vi "AlliGator Clip Decay for Fit.vi"(8 "Error In":errorcluster, 9 "Min Decay Percentile (0)":dbl, 10 "Max Decay Percentile (1)":dbl=1.0, 11 "Decay in":cluster{"t Array":dbl[], "Value Array":dbl[]}) -> (0 "Error Out":errorcluster, 1 "Index Min":i32, 2 "Index Max":i32, 3 "Clipped Decay out":cluster{"t Array":dbl[], "Value Array":dbl[]}, 4 "# Points":i32)   [LabVIEW 2021, in "AlliGator Decay Analysis.lvlib" / "AlliGator Decay Fit.lvlib"]
doc: "Clips the decay according to the <B>Min</B> and <B>Max Decay Percentile</B> parameters provided.\n\nIf the decay range is [I_min, I_max] and the decay percentiles are (f_min, f_max) in [0, 1], we look for:\n\n- starting from the location of the maximum (presumably the peak location) and moving forward, the point at which:\n\nI_i < I_min + f_max*(I_max - I_min) = F_max\n\n- starting from the last point and moving baclwards, the point at which:\n\nI_i > I_min + f_min*(I_max - I_min) = F_min"
uses:
  AlliGator Decay Fit.lvlib
panel:
  out "XY Graph":cluster{"t Array":dbl[], "Value Array":dbl[]}[](graph)
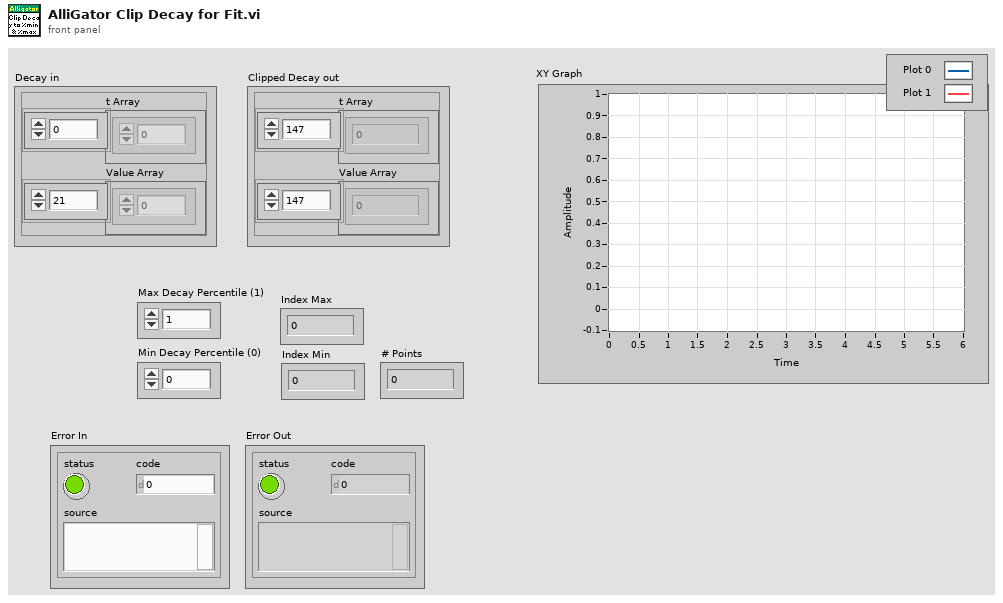
[diagram p1: front panel]
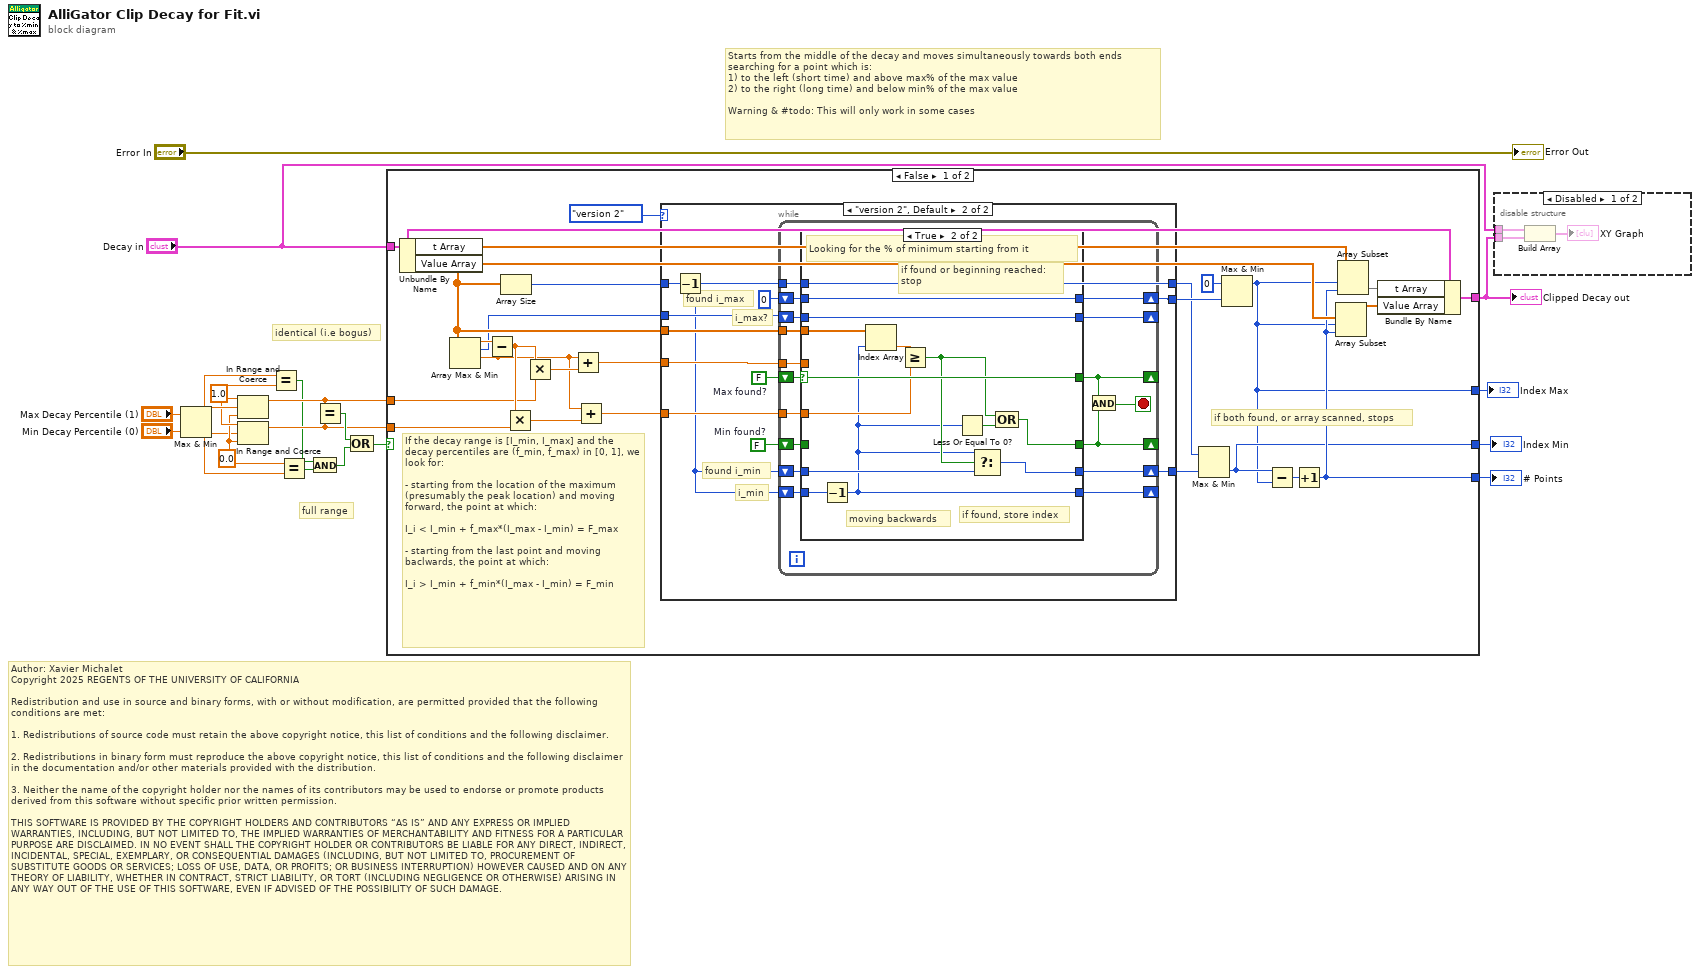
[diagram p0: block diagram]
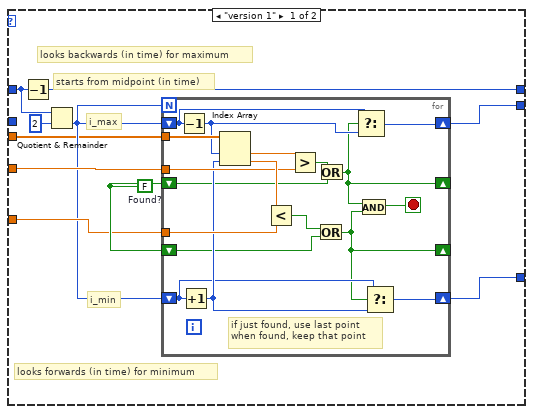
[diagram p2: hidden frame]
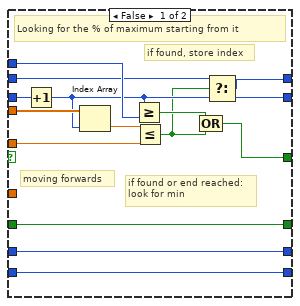
[diagram p3: hidden frame]
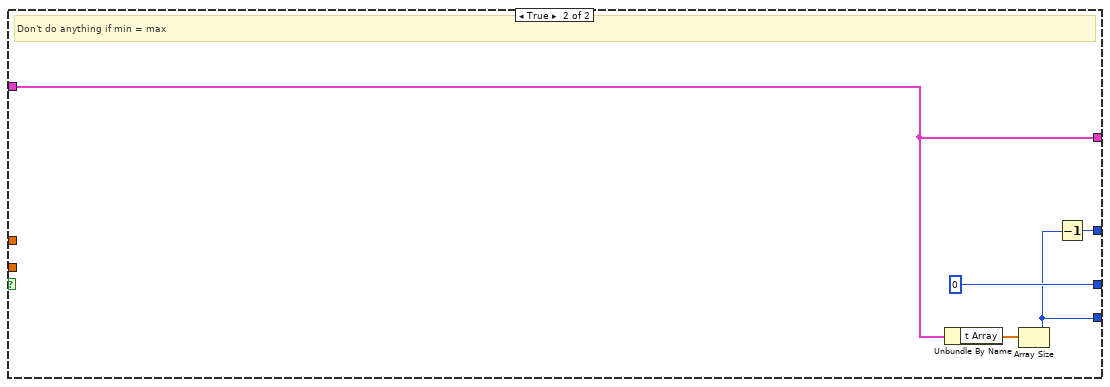
[diagram p4: hidden frame]
diagram:
  w7 = 1.0 ("upper limit")
  w6 = 0.0 ("lower limit")
  # "Author: Xavier Michalet\nCopyright 2025 REGENTS OF THE UNIVERSITY OF CALIFORNIA\n\nRedistribution and use in source and binary forms, with or without modification, are permitted provided that the following conditions are met:\n\n1. Redistributions of source code must retain the above copyright notice, this list of conditions and the following disclaimer.\n\n2. Redistributions in binary form must reproduce the above copyright notice, this list of conditions and the following disclaimer in the documentation and/or other materials provided with the distribution.\n\n3. Neither the name of the copyright holder nor the names of its contributors may be used to endorse or promote products derived from this software without specific prior written permission.\n\nTHIS SOFTWARE IS PROVIDED BY THE COPYRIGHT HOLDERS AND CONTRIBUTORS “AS IS” AND ANY EXPRESS OR IMPLIED WARRANTIES, INCLUDING, BUT NOT LIMITED TO, THE IMPLIED WARRANTIES OF MERCHANTABILITY AND FITNESS FOR A PARTICULAR PURPOSE ARE DISCLAIMED. IN NO EVENT SHALL THE COPYRIGHT HOLDER OR CONTRIBUTORS BE LIABLE FOR ANY DIRECT, INDIRECT, INCIDENTAL, SPECIAL, EXEMPLARY, OR CONSEQUENTIAL DAMAGES (INCLUDING, BUT NOT LIMITED TO, PROCUREMENT OF SUBSTITUTE GOODS OR SERVICES; LOSS OF USE, DATA, OR PROFITS; OR BUSINESS INTERRUPTION) HOWEVER CAUSED AND ON ANY THEORY OF LIABILITY, WHETHER IN CONTRACT, STRICT LIABILITY, OR TORT (INCLUDING NEGLIGENCE OR OTHERWISE) ARISING IN ANY WAY OUT OF THE USE OF THIS SOFTWARE, EVEN IF ADVISED OF THE POSSIBILITY OF SUCH DAMAGE."
  # "identical (i.e bogus)"
  # "full range"
  # "Starts from the middle of the decay and moves simultaneously towards both ends\nsearching for a point which is:\n1) to the left (short time) and above max% of the max value\n2) to the right (long time) and below min% of the max value\n\nWarning & #todo: This will only work in some cases"
  n1 = Max & Min(x="Max Decay Percentile (1)", y="Min Decay Percentile (0)") -> (max(x,y)=w8:dbl, min(x,y)=w5:dbl)
  n2 = In Range and Coerce(upper limit=w7, x=w8, lower limit=w6) -> (coerced(x)=w9:dbl)  [unwired: 1 out]
  n3 = In Range and Coerce(upper limit=w7, x=w5, lower limit=w6) -> (coerced(x)=w10:dbl)  [unwired: 1 out]
  n4 = Equal?(x=w8, y=w7) -> (x = y?=w2:bool)
  n5 = Equal?(x=w6, y=w5) -> (x = y?=w3:bool)
  n6 = And(x=w2, y=w3) -> (x .and. y?=w1:bool)
  n7 = Equal?(x=w9, y=w10) -> (x = y?=w11:bool)
  n8 = Compound Arithmetic op=OR(w11, w1) -> (w4:bool)
  n9 = case shown="False" w4 {
    tunnel: "Decay in" -> [w32 w133]
    tunnel: [w31 w133] -> w17
    tunnel: w9 -> [w26 _]
    tunnel: w10 -> [w25 _]
    tunnel: [w24 w130] -> w16
    tunnel: [w23 0] -> w15
    tunnel: [w22 w129] -> w14
    frame False {
      # "If the decay range is [I_min, I_max] and the decay percentiles are (f_min, f_max) in [0, 1], we look for:\n\n- starting from the location of the maximum\n(presumably the peak location) and moving \nforward, the point at which:\n\nI_i < I_min + f_max*(I_max - I_min) = F_max\n\n- starting from the last point and moving\nbaclwards, the point at which:\n\nI_i > I_min + f_min*(I_max - I_min) = F_min"
      # "if both found, or array scanned, stops"
      n10 = Unbundle By Name(w32) -> ("t Array"=w38:dbl[], "Value Array"=w35:dbl[])
      n11 = Array Max & Min(array=w35) -> (max value=w45:dbl, max index (indices)=w20:i32, min value=w41:dbl)  [unwired: 1 out]
      n12 = Subtract(x=w45, y=w41) -> (x-y=w44:dbl)
      n13 = Array Size(array=w35) -> (size(s)=w30:i32)
      n14 = Multiply(x=w44, y=w25) -> (x*y=w42:dbl)
      n15 = Multiply(x=w44, y=w26) -> (x*y=w43:dbl)
      n16 = Add(x=w41, y=w43) -> (x+y=w40:dbl)
      n17 = Add(x=w41, y=w42) -> (x+y=w39:dbl)
      n18 = case shown="\"version 2\", Default" enum16{"version 1", "version 2"}."version 2" {
        tunnel: w40 -> [w53 w83]
        tunnel: w39 -> [w52 w82]
        tunnel: w35 -> [w50 w81]
        tunnel: [w49 w76] -> w34
        tunnel: w30 -> [w48 w80]
        tunnel: [w47 w75] -> w29
        tunnel: [w46 w74] -> w28
        tunnel: w20 -> [_ w78]
        frame "version 1" {
          w55 = FALSE  # Found?
          # "looks forwards (in time) for minimum"
          # "looks backwards (in time) for maximum"
          # "starts from midpoint (in time)"
          # "i_min"
          # "i_max"
          n19 = Decrement(x=w48) -> (x-1=w46:i32)
          n20 = Quotient & Remainder(x=w48, y=2) -> (floor(x/y)=w51:i32)  [unwired: 1 out]
          n21 = for {
            N: w51 -> [_]
            shift-right: [w66] -> w49
            shift-left: w51 -> [w67]
            shift-right: [w62] -> w47
            shift-left: w51 -> [w61]
            tunnel: w53 -> [w69]
            tunnel: w52 -> [w71]
            tunnel: w50 -> [w73]
            shift-right: [w57] -> _
            shift-left: w55 -> [w60]
            shift-right: [w56] -> _
            shift-left: w55 -> [w59]
            stop <- w58 stop-if-true
            # "if just found, use last point\nwhen found, keep that point"
            n22 = Decrement(x=w67) -> (x-1=w65:i32)
            n23 = Increment(x=w61) -> (x+1=w63:i32)
            n24 = Index Array(array=w73, index #1=w65, index #2=w63) -> (element #1=w70:dbl, element #2=w72:dbl)
            n25 = Less?(x=w72, y=w71) -> (x < y?=w64:bool)
            n26 = Greater?(x=w70, y=w69) -> (0:w68:bool)
            n27 = Or(x=w64, y=w59) -> (x .or. y?=w56:bool)
            n28 = Or(x=w68, y=w60) -> (x .or. y?=w57:bool)
            n29 = Select(t=w67, s=w57, f=w65) -> (s? t:f=w66:i32)
            n30 = And(x=w57, y=w56) -> (x .and. y?=w58:bool)
            n31 = Select(t=w61, s=w56, f=w63) -> (s? t:f=w62:i32)
          }
        }
        frame "version 2", Default {
          w79 = FALSE  # Min found?
          w84 = FALSE  # Max found?
          # "found i_min"
          # "found i_max"
          # "i_min"
          # "i_max?"
          n32 = Decrement(x=w80) -> (x-1=w74:i32)
          n33 = while {
            shift-right: [w97] -> _
            shift-left: w78 -> [w98]
            shift-right: [w96] -> _
            shift-left: w74 -> [w95]
            tunnel: w83 -> [w99]
            tunnel: w82 -> [w100]
            tunnel: w81 -> [w101]
            shift-right: [w88] -> _
            shift-left: w84 -> [w94]
            shift-right: [w92] -> _
            shift-left: w79 -> [w93]
            tunnel: w74 -> [w91]
            shift-right: [w89] -> w76
            shift-left: 0 -> [w90]
            shift-right: [w85] -> w75
            shift-left: w74 -> [w86]
            stop <- w87 stop-if-true
            n34 = case shown="True" w94 {
              selector: w94 -> [_ w125]
              tunnel: w101 -> [w115 w128]
              tunnel: w100 -> [_ w124]
              tunnel: w99 -> [w113 _]
              tunnel: w98 -> [w112 w126]
              tunnel: [w108 w126] -> w97
              tunnel: [w103 w117] -> w96
              tunnel: w95 -> [w103 w123]
              tunnel: w93 -> [w111 _]
              tunnel: [w104 w125] -> w88
              tunnel: [w111 w121] -> w92
              tunnel: w91 -> [w110 _]
              tunnel: w90 -> [w109 w122]
              tunnel: [w107 w122] -> w89
              tunnel: w86 -> [w102 w119]
              tunnel: [w102 w120] -> w85
              frame False {
                # "moving forwards"
                # "if found, store index"
                # "if found or end reached:\nlook for min"
                # "Looking for the % of maximum starting from it"
                n35 = Increment(x=w112) -> (x+1=w108:i32)
                n36 = Index Array(array=w115, index=w108) -> (element=w114:dbl)
                n37 = Greater Or Equal?(x=w108, y=w110) -> (x >= y?=w106:bool)
                n38 = Less Or Equal?(x=w114, y=w113) -> (x <= y?=w105:bool)
                n39 = Compound Arithmetic op=OR(w106, w105) -> (w104:bool)
                n40 = Select(t=w109, s=w105, f=w108) -> (s? t:f=w107:i32)
              }
              frame True {
                # "if found, store index"
                # "moving backwards"
                # "if found or beginning reached:\nstop"
                # "Looking for the % of minimum starting from it"
                n41 = Decrement(x=w123) -> (x-1=w117:i32)
                n42 = Index Array(array=w128, index=w117) -> (element=w127:dbl)
                n43 = Greater Or Equal?(x=w127, y=w124) -> (x >= y?=w118:bool)
                n44 = Less Or Equal To 0?(x=w117) -> (x <= 0?=w116:bool)
                n45 = Select(t=w117, s=w118, f=w119) -> (s? t:f=w120:i32)
                n46 = Compound Arithmetic op=OR(w118, w116) -> (w121:bool)
              }
            }
            n47 = And(x=w88, y=w92) -> (x .and. y?=w87:bool)
          }
        }
      }
      n48 = Max & Min(x=w28, y=w29) -> (min(x,y)=w23:i32)  [unwired: 1 out]
      n49 = Max & Min(x=0, y=w34) -> (max(x,y)=w22:i32)  [unwired: 1 out]
      n50 = Subtract(x=w23, y=w22) -> (x-y=w36:i32)
      n51 = Increment(x=w36) -> (x+1=w24:i32)
      n52 = Array Subset(array=w35, index=w22, length=w24) -> (w33:dbl[])
      n53 = Array Subset(array=w38, index=w22, length=w24) -> (w37:dbl[])
      n54 = Bundle By Name(cluster=w32, "t Array"=w37, "Value Array"=w33) -> (w31:cluster{"t Array":dbl[], "Value Array":dbl[]})
    }
    frame True {
      # "Don't do anything if min = max"
      n55 = Unbundle By Name(w133) -> ("t Array"=w132:dbl[])
      n56 = Array Size(array=w132) -> (size(s)=w130:i32)
      n57 = Decrement(x=w130) -> (x-1=w129:i32)
    }
  }
  "Clipped Decay out" <- w17
  "Index Max" <- w14
  "Index Min" <- w15
  "# Points" <- w16
  n58 = disable-structure shown="Disabled" {
    disable-tunnel: "Decay in" -> [w136 _]
    disable-tunnel: w17 -> [w135 _]
    frame Disabled {
      n59 = Build Array(w136, w135) -> (→"XY Graph":cluster{"t Array":dbl[], "Value Array":dbl[]}[])
    }
    frame Enabled {
    }
  }
  "Error Out" <- "Error In"
